vi "Read Photodiodes.vi"(1 "Buffer size (samples per channel)":u32=2000384, 2 "Time to sample (seconds)":dbl=2.0, 3 "Sample Rate (Hz)":dbl=1000000.0 format="%0.2f", 4 "Diode tdms path":path) -> (0 "error out":errorcluster)   [LabVIEW 2018]
uses:
  <vilib>/DAQmx/read.llb/DAQmx Read (Analog 1D Wfm NChan NSamp).vi
  <vilib>/DAQmx/create/channels.llb/DAQmx Create Channel (AI-Voltage-Basic).vi
  <vilib>/DAQmx/configure/timing.llb/DAQmx Timing (Sample Clock).vi
  <vilib>/DAQmx/configure/task.llb/DAQmx Configure Logging (TDMS).vi
  <vilib>/DAQmx/miscellaneous.llb/DAQmx Fill In Error Info.vi
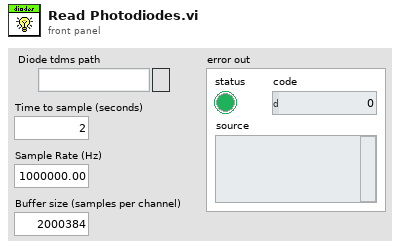
[diagram p1: front panel]
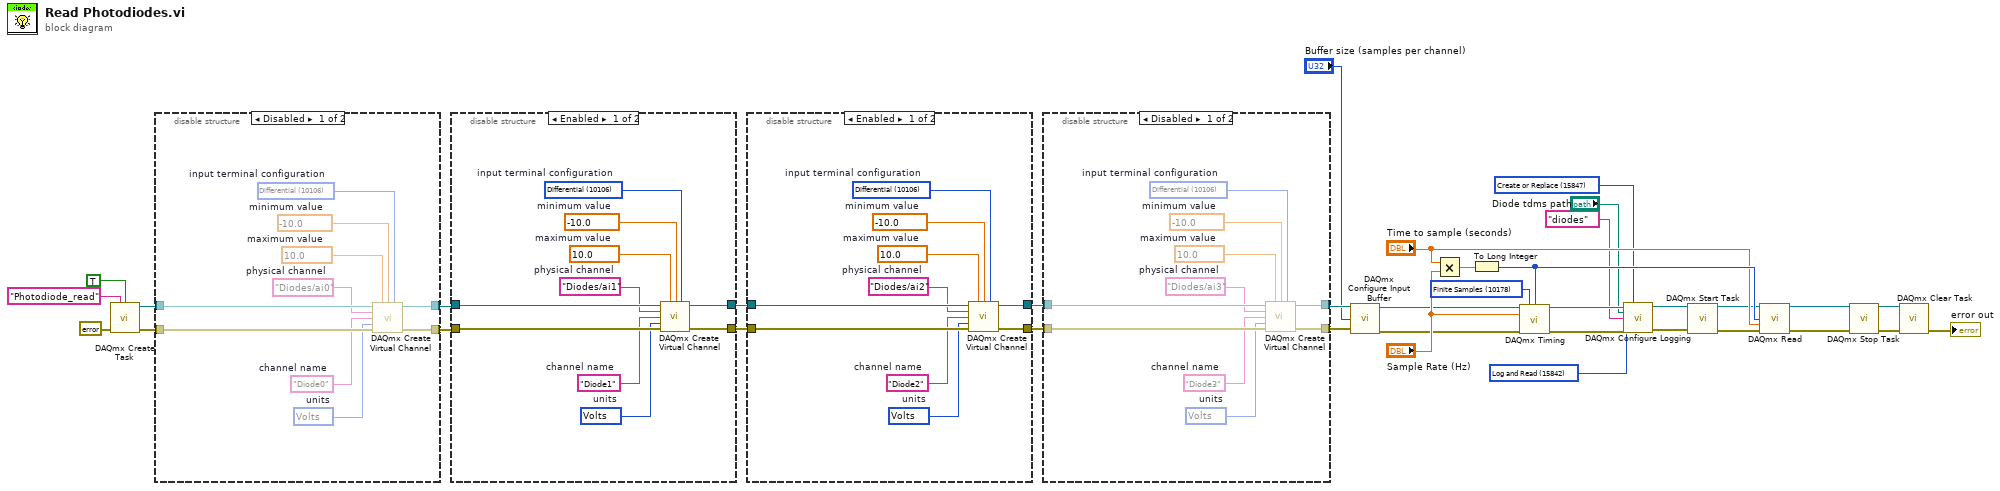
[diagram p0: block diagram]
diagram:
  w6 = 15847 items=["Open"=10437, "Open or Create"=15846, "Create or Replace"=15847, "Create"=15848] ("operation")
  w7 = 15842 items=["Off"=10231, "Log"=15844, "Log and Read"=15842] ("logging mode")
  w32 = 10178 items=["Finite Samples"=10178, "Continuous Samples"=10123, "Hardware Timed Single Point"=12522] ("sample mode")
  n1 = call <vilib>:"DAQmx Create Task.vi"("new task name"="Photodiode_read", "auto cleanup"=TRUE, "error in"=errorcluster {"status"=FALSE, "code"=0, "source"=""}) -> ("task out"=w34:refnum<k21>, "error out"=w36:errorcluster)  [unwired: 11 in]
  n2 = disable-structure shown="Disabled" {
    disable-tunnel: w36 -> [w46 w47]
    disable-tunnel: w34 -> [w45 w48]
    disable-tunnel: [w41 w47] -> w31
    disable-tunnel: [w37 w48] -> w30
    frame Disabled {
      w38 = 10106 items=["default"=-1, "RSE"=10083, "NRSE"=10078, "Differential"=10106, "Pseudodifferential"=12529]  # input terminal configuration
      w39 = 10348 items=["Volts"=10348, "From Custom Scale"=10065]  # units
      w40 = "Diode0"  # channel name
      w42 = -10.0  # minimum value
      w43 = 10.0  # maximum value
      w44 = "Diodes/ai0"  # physical channel
      n3 = call-poly <vilib>:"DAQmx Create Virtual Channel.vi"("task in"=w45, "maximum value"=w43, "minimum value"=w42, "input terminal configuration"=w38, "physical channels"=w44, "name to assign"=w40, "units"=w39, "error in"=w46) -> ("task out"=w37:refnum<k21>, "error out"=w41:errorcluster)  [unwired: 6 in]
    }
    frame Enabled {
    }
  }
  n4 = disable-structure shown="Enabled" {
    disable-tunnel: w31 -> [w58 w59]
    disable-tunnel: w30 -> [w57 w60]
    disable-tunnel: [w53 w59] -> w26
    disable-tunnel: [w49 w60] -> w25
    frame Enabled {
      w50 = 10106 items=["default"=-1, "RSE"=10083, "NRSE"=10078, "Differential"=10106, "Pseudodifferential"=12529]  # input terminal configuration
      w51 = 10348 items=["Volts"=10348, "From Custom Scale"=10065]  # units
      w52 = "Diode1"  # channel name
      w54 = -10.0  # minimum value
      w55 = 10.0  # maximum value
      w56 = "Diodes/ai1"  # physical channel
      n5 = call-poly <vilib>:"DAQmx Create Virtual Channel.vi"("task in"=w57, "maximum value"=w55, "minimum value"=w54, "input terminal configuration"=w50, "physical channels"=w56, "name to assign"=w52, "units"=w51, "error in"=w58) -> ("task out"=w49:refnum<k21>, "error out"=w53:errorcluster)  [unwired: 6 in]
    }
    frame Disabled {
    }
  }
  n6 = disable-structure shown="Enabled" {
    disable-tunnel: w26 -> [w70 w72]
    disable-tunnel: w25 -> [w69 w71]
    disable-tunnel: [w68 w72] -> w24
    disable-tunnel: [w67 w71] -> w23
    frame Enabled {
      w61 = 10106 items=["default"=-1, "RSE"=10083, "NRSE"=10078, "Differential"=10106, "Pseudodifferential"=12529]  # input terminal configuration
      w62 = 10348 items=["Volts"=10348, "From Custom Scale"=10065]  # units
      w63 = "Diode2"  # channel name
      w64 = -10.0  # minimum value
      w65 = 10.0  # maximum value
      w66 = "Diodes/ai2"  # physical channel
      n7 = call-poly <vilib>:"DAQmx Create Virtual Channel.vi"("task in"=w69, "maximum value"=w65, "minimum value"=w64, "input terminal configuration"=w61, "physical channels"=w66, "name to assign"=w63, "units"=w62, "error in"=w70) -> ("task out"=w67:refnum<k21>, "error out"=w68:errorcluster)  [unwired: 6 in]
    }
    frame Disabled {
    }
  }
  n8 = disable-structure shown="Disabled" {
    disable-tunnel: [w82 w83] -> w2
    disable-tunnel: [w81 w84] -> w5
    disable-tunnel: w24 -> [w80 w84]
    disable-tunnel: w23 -> [w79 w83]
    frame Disabled {
      w74 = 10106 items=["default"=-1, "RSE"=10083, "NRSE"=10078, "Differential"=10106, "Pseudodifferential"=12529]  # input terminal configuration
      w75 = 10348 items=["Volts"=10348, "From Custom Scale"=10065]  # units
      w73 = "Diode3"  # channel name
      w76 = -10.0  # minimum value
      w77 = 10.0  # maximum value
      w78 = "Diodes/ai3"  # physical channel
      n9 = call-poly <vilib>:"DAQmx Create Virtual Channel.vi"("task in"=w79, "maximum value"=w77, "minimum value"=w76, "input terminal configuration"=w74, "physical channels"=w78, "name to assign"=w73, "units"=w75, "error in"=w80) -> ("task out"=w82:refnum<k21>, "error out"=w81:errorcluster)  [unwired: 6 in]
    }
    frame Enabled {
    }
  }
  n10 = call <vilib>:"DAQmx Configure Input Buffer.vi"("task/channels in"=w2, "buffer size (in samples per channel)"="Buffer size (samples per channel)", "error in"=w5) -> ("task out"=w3:refnum<k21>, "error out"=w4:errorcluster)  [unwired: 11 in]
  n11 = Multiply(x="Time to sample (seconds)", y="Sample Rate (Hz)") -> (x*y=w27:dbl)
  n12 = To Long Integer(number=w27) -> (32bit integer=w21:i32)
  n13 = call-poly <vilib>:"DAQmx Timing.vi"("task/channels in"=w3, "sample mode"=w32, "samples per channel"=w21, "rate"="Sample Rate (Hz)", "error in"=w4) -> ("task out"=w13:refnum<k21>, "error out"=w12:errorcluster)  [unwired: 9 in]
  n14 = call-poly <vilib>:"DAQmx Configure Logging.vi"("task/channels in"=w13, "operation"=w6, "file path"="Diode tdms path", "group name"="diodes" ("Measurement type"), "logging mode"=w7, "error in"=w12) -> ("task out"=w10:refnum<k21>, "error out"=w11:errorcluster)  [unwired: 8 in]
  n15 = call <vilib>:"DAQmx Start Task.vi"("task/channels in"=w10, "error in"=w11) -> ("task out"=w18:refnum<k21>, "error out"=w19:errorcluster)  [unwired: 12 in]
  n16 = call-poly <vilib>:"DAQmx Read.vi"("task/channels in"=w18, "number of samples per channel"=w21, "timeout"="Time to sample (seconds)", "error in"=w19) -> ("task out"=w17:refnum<k21>, "error out"=w14:errorcluster)  [unwired: 9 in, 1 out]
  n17 = call <vilib>:"DAQmx Stop Task.vi"("task/channels in"=w17, "error in"=w14) -> ("task out"=w16:refnum<k21>, "error out"=w15:errorcluster)  [unwired: 12 in]
  n18 = call <vilib>:"DAQmx Clear Task.vi"("task in"=w16, "error in"=w15) -> ("error out"=→"error out":errorcluster)  [unwired: 13 in]
